vi "Run.vi"(8 "error in":errorcluster, 10 "ID":string, 11 "Client in":refnum<class "Client.lvclass">) -> (0 "error out":errorcluster, 3 "Client out":refnum<class "Client.lvclass">)   [LabVIEW 2014, in "Client.lvclass"]
uses:
  Client.lvclass
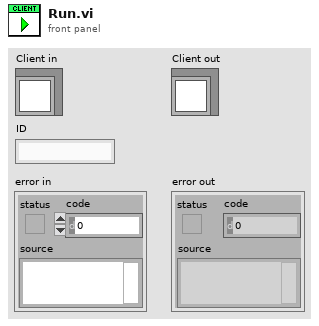
[diagram p1: front panel]
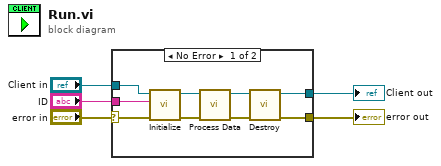
[diagram p0: block diagram]
diagram:
  n1 = case shown="No Error" "error in" {
    selector: "error in" -> [w6 w16]
    tunnel: [w9 w16] -> w4
    tunnel: [w12 w15] -> w2
    tunnel: "Client in" -> [w8 w15]
    tunnel: "ID" -> [w7 _]
    frame No Error {
      n2 = call-dynamic "Initialize.vi"("error in"=w6, "ID"=w7, "Client in"=w8) -> ("error out"=w11:errorcluster, "Client out"=w14:refnum<class "Client.lvclass">)  [unwired: 7 in]
      n3 = call-dynamic "Process Data.vi"("error in"=w11, "Client in"=w14) -> ("error out"=w10:errorcluster, "Client out"=w13:refnum<class "Client.lvclass">)  [unwired: 8 in]
      n4 = call-dynamic "Destroy.vi"("error in"=w10, "Client in"=w13) -> ("error out"=w9:errorcluster, "Client out"=w12:refnum<class "Client.lvclass">)  [unwired: 8 in]
    }
    frame Error {
    }
  }
  "error out" <- w4
  "Client out" <- w2
